vi "readPosistionFirgelli.vi"(8 "error in (no error)":errorcluster, 11 "handleIn":u32 format="%x") -> (0 "error out":errorcluster, 2 "pDataOut":u8[](array[numeric]), 3 "handleOut":u32 format="%x")   [LabVIEW 2016]
doc: "(Distance / Stroke) × 1023\n\nFor example, to half way extend(25mm) a 50mm actuator, send 512. (The calculated value is rounded to a whole number).\n\n\nWritten by: Complete Automated Solutions\nwww.CompleteAutomatedSolutions.com"
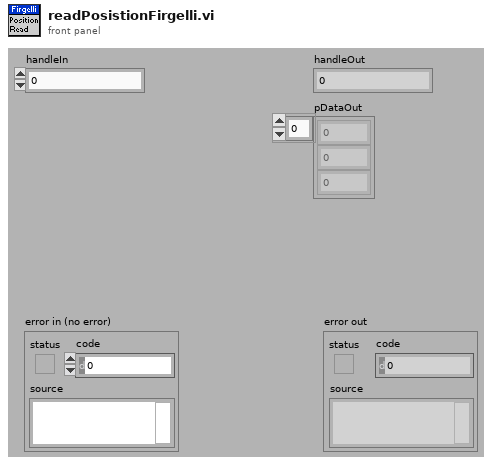
[diagram p1: front panel]
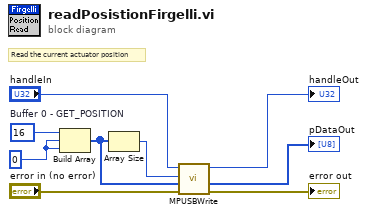
[diagram p0: block diagram]
diagram:
  w4 = u8 0 ("element")
  w5 = u8 16  # Buffer 0 - GET_POSITION
  # "Read the current actuator position"
  n1 = Build Array(w5, w4, w4) -> (w2:u8[])
  n2 = Array Size(array=w2) -> (size(s)=w3:i32)
  n3 = call "MPUSBWrite.vi"("error in (no error)"="error in (no error)", "pDataIn"=w2, "dwLen"=w3, "handleIn"="handleIn") -> ("error out"=→"error out":errorcluster, "pDataOut"=→"pDataOut":u8[], "handleOut"=→"handleOut":u32)  [unwired: 1 in, 4 out]
